vi "1-DOF_Helicopter.vi"() -> ()   [LabVIEW 2021]
uses:
  <vilib>/MakerHub/LINX/Public/Sensors/Accelerometer/MPU60X0/GyroFullScaleRanges.ctl
  <vilib>/MakerHub/LINX/Public/Sensors/Accelerometer/MPU60X0/DeviceAddresses.ctl
  <vilib>/MakerHub/LINX/Public/Peripherals/Digital/Digital Write 1 Chan.vi
  <vilib>/MakerHub/LINX/Public/Peripherals/PWM/PWM Set Duty Cycle 1 Chan.vi
  <vilib>/MakerHub/LINX/Public/Peripherals/Digital/Digital Write N Chans.vi
  <vilib>/MakerHub/LINX/Private/Local IO/LinxDigitalWrite.vi
  <vilib>/MakerHub/LINX/Public/Utilities/Check Channel.vi
  <vilib>/MakerHub/LINX/Public/Utilities/Open Serial.vi
  <vilib>/MakerHub/LINX/Private/Utilties/Generate Error.vi
  <vilib>/MakerHub/LINX/Public/Peripherals/PWM/PWM Set Duty Cycle N Chans.vi
  <vilib>/MakerHub/LINX/Public/Sensors/Accelerometer/MPU60X0/MPU60X0.lvlib
  <vilib>/MakerHub/LINX/LMH-LINX.lvlib
panel:
  out "PWM":ext
  in  "Serial Port":refnum<visa-resource-name>="N/A"
  out "milliseconds  3":ext
  in  "milliseconds  2":ext=1.0
  in  "kp(x)":ext
  in  "kd(x)":ext
  out "e(x)":ext
  out "x Angle":ext(graph)
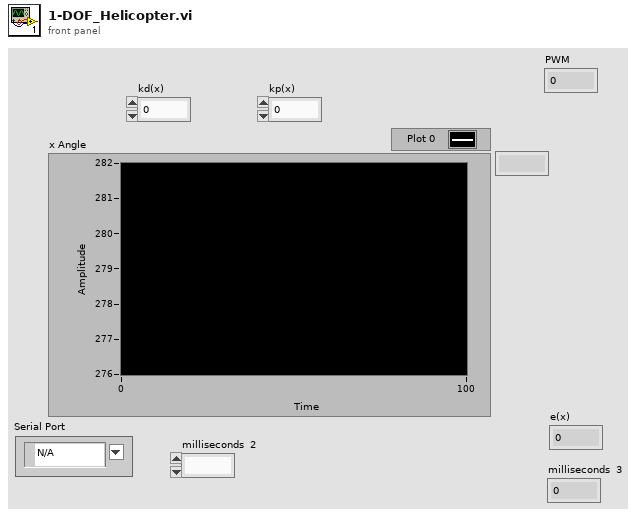
[diagram p1: front panel]
types:
  T1 = typedef "LMH-LINX.lvlib/MPU60X0.lvlib/DeviceAddresses.ctl" = enum16{"0x68", "0x69"}
  T2 = typedef "LMH-LINX.lvlib/MPU60X0.lvlib/GyroFullScaleRanges.ctl" = enum8{"±250 °/s", "±500 °/s", "±1000 °/s", "±2000 °/s"}
  T3 = typedef "LMH-LINX.lvlib/LINX Ref.ctl" = cluster{"IO":T4, "Interface":T5, "LINX Device Config":T6}
  T4 = typedef "LMH-LINX.lvlib/Platform.ctl" = enum16{"Remote", "Local"}
  T5 = typedef "LMH-LINX.lvlib/Interface.ctl" = enum16{"Serial", "TCP"}
  T6 = typedef "LMH-LINX.lvlib/Device.lvlib/LINX Device Config.ctl" = cluster{"Interface":T5, "COM Port":refnum<visa-resource-name>, "TCP Configuration":T7, "Device Family":u8, "Device ID":u8, "Device Name":string, "TCP Ref":refnum<k5>, "Channels":T8}
  T7 = typedef "LMH-LINX.lvlib/Device.lvlib/TCP Config.ctl" = cluster{"IP Address":string, "Port":u16}
  T8 = typedef "LMH-LINX.lvlib/Channels.ctl" = cluster{"DI":u8[], "DO":u8[], "AI":u8[], "AO":u8[], "PWM":u8[], "QE":u8[], "UART":u8[], "I2C 2":u8[], "SPI":u8[], "CAN":u8[], "Servo":u8[], "AI Ref (V)":dbl, "AI Resolution (Bits)":u8, "AO Ref (V)":dbl, "AO Resolution (Bits)":u8}
  T9 = cluster{"X Axis":i16, "Y Axis":i16, "Z Axis":i16}
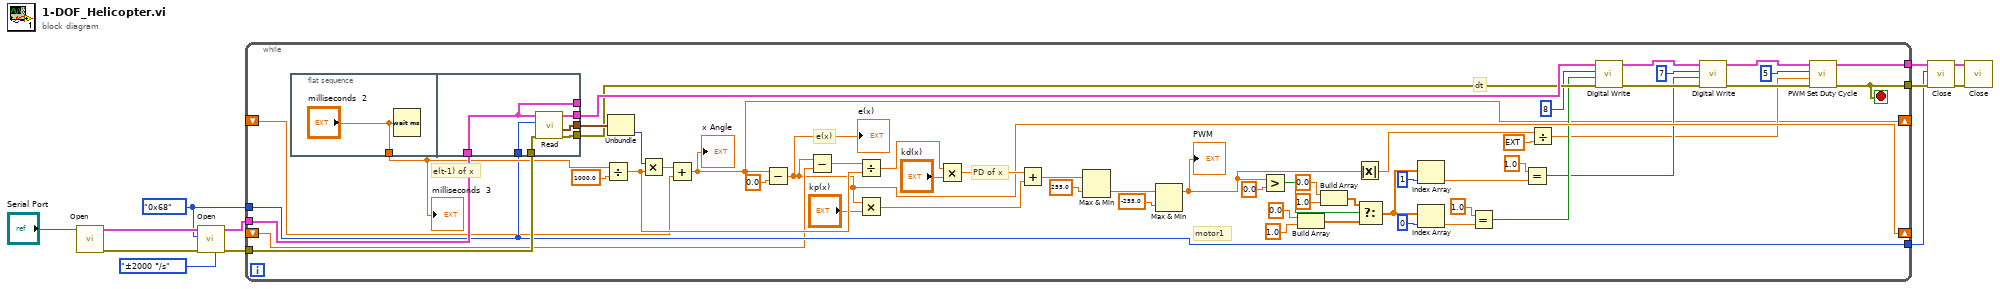
[diagram p0: block diagram]
diagram:
  w2 = DeviceAddresses."0x68" ("I2C Slave Address")
  n1 = call-poly <vilib>:"Open.vi"("Serial Port"="Serial Port") -> ("Error Out"=w12:errorcluster, "LINX Resource"=w11:T3)  [unwired: 8 in, 1 out]
  n2 = call <vilib>:"Open.vi"("Gyro Full Scale Range"=GyroFullScaleRanges."±2000 °/s", "Error In"=w12, "I2C Slave Address"=w2, "LINX Resource"=w11) -> ("Error Out"=w9:errorcluster, "LINX Resource"=w10:T3)  [unwired: 6 in]
  n3 = while {
    tunnel: w10 -> [w59]
    tunnel: w9 -> [w58]
    tunnel: [w22] -> w4
    tunnel: [w13] -> w3
    tunnel: w2 -> [w55]
    tunnel: [w55] -> w1
    shift-right: [w53] -> _
    shift-left: _ -> [w54]
    shift-right: [w15] -> _
    shift-left: _ -> [w16]
    stop <- w13 stop-if-true
    # "motor1"
    # "PD of x"
    # "e(x)"
    # "dt"
    # "e(t-1) of x"
    n4 = flat-sequence {
      tunnel: ["milliseconds  2"] -> w56
      tunnel: [w75] -> w23
      tunnel: [w74] -> w57
      tunnel: [w73] -> w24
      tunnel: [w71] -> _
      tunnel: w55 -> [w72]
      tunnel: w59 -> [w71]
      tunnel: w58 -> [w70]
      frame #0 {
        n5 = Wait (ms)(milliseconds to wait="milliseconds  2") -> ()  [unwired: 1 out]
      }
      frame #1 {
        n6 = call <vilib>:"Read.vi"("Error In"=w70, "I2C Slave Address"=w72, "LINX Resource"=w71) -> ("Error Out"=w75:errorcluster, "Gyro  Data (dps)"=w74:T9, "LINX Resource"=w73:T3)  [unwired: 4 in, 2 out]
      }
    }
    n7 = Divide(x=w56, y=1000.0) -> (x/y=w65:ext)
    n8 = Unbundle(w57) -> ("Z Axis"=w14:i16)  [unwired: 2 out]
    n9 = Multiply(x=w14, y=w65) -> (x*y=w17:ext)
    n10 = Add(x=w17, y=w16) -> (x+y=w15:ext)
    "x Angle" <- w15
    n11 = Subtract(x=w15, y=0.0) -> (x-y=w53:ext)
    "e(x)" <- w53
    n12 = Subtract(x=w53, y=w54) -> (x-y=w66:ext)
    n13 = Divide(x=w66, y=w65) -> (x/y=w64:ext)
    n14 = Multiply(x=w53, y="kp(x)") -> (x*y=w60:ext)
    n15 = Multiply(x=w64, y="kd(x)") -> (x*y=w61:ext)
    n16 = Add(x=w61, y=w60) -> (x+y=w31:ext)
    n17 = Max & Min(x=w31, y=255.0) -> (min(x,y)=w52:ext)  [unwired: 1 out]
    n18 = Max & Min(x=w52, y=-255.0) -> (max(x,y)=w48:ext)  [unwired: 1 out]
    "PWM" <- w48
    n19 = Greater?(x=w48, y=0.0) -> (0:w45:bool)
    n20 = Build Array(0.0 ("element"), 1.0 ("element")) -> (w43:dbl[])
    n21 = Build Array(0.0 ("element"), 1.0 ("element")) -> (w44:dbl[])
    n22 = Absolute Value(x=w48) -> (abs(x)=w47:ext)
    n23 = Select(t=w44, s=w45, f=w43) -> (s? t:f=w32:dbl[])
    n24 = Index Array(array=w32, index=1) -> (element=w38:dbl)
    n25 = Index Array(array=w32, index=0) -> (element=w37:dbl)
    n26 = Equal?(x=1.0, y=w37) -> (x = y?=w20:bool)
    n27 = Equal?(x=1.0, y=w38) -> (x = y?=w19:bool)
    n28 = Divide(x=w47, y=ext 255.0) -> (x/y=w18:ext)
    n29 = call-poly <vilib>:"Digital Write.vi"("Error In"=w23, "Output Value"=w20, "DO Channel"=u8 8, "LINX Resource"=w24) -> ("Error Out"=w29:errorcluster, "LINX Resource"=w27:T3)  [unwired: 6 in]
    n30 = call-poly <vilib>:"Digital Write.vi"("Error In"=w29, "Output Value"=w19, "DO Channel"=u8 7, "LINX Resource"=w27) -> ("Error Out"=w25:errorcluster, "LINX Resource"=w26:T3)  [unwired: 6 in]
    n31 = call-poly <vilib>:"PWM Set Duty Cycle.vi"("Error In"=w25, "Duty Cycle (0-1)"=w18, "PWM Channel"=u8 5, "LINX Resource"=w26) -> ("Error Out"=w13:errorcluster, "LINX Resource"=w22:T3)  [unwired: 6 in]
    "milliseconds  3" <- w56
  }
  n32 = call <vilib>:"Close.vi"("Error In"=w3, "I2C Slave Address (0)"=w1, "LINX Resource"=w4) -> ("Error Out"=w5:errorcluster, "LINX Resource"=w6:T3)  [unwired: 7 in]
  n33 = call <vilib>:"Close.vi"("Error In"=w5, "LINX Resource"=w6) -> ()  [unwired: 9 in, 1 out]
